vi "备用系数复合写入.vi"(8 "备用系数":cluster{"上限":dbl, "下限":dbl, "范围":dbl}, 9 "量程下拉列表":enum16{"低量程", "高量程"}(ring), 10 "测量模式":T1(ring), 11 "参数下拉列表":u16(ring) items=["总氮"=2]) -> ()   [LabVIEW 2016, in "斯坦道通用流路CODmn.lvlib"]
uses:
  <vilib>/Utility/miscctls.llb/LVPointTypeDef.ctl
panel:
  in  "读取":bool
  in  "一键写入":bool=TRUE
  out "连接的字符串":string
  in  "关闭":bool
  in  "写入":bool
  # "请选择要写入的参数"
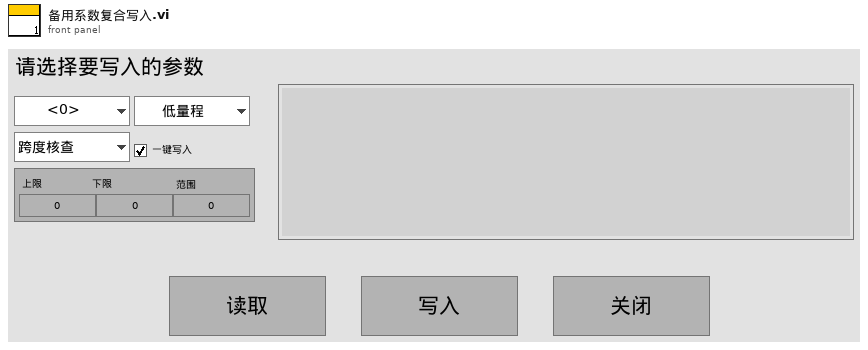
[diagram p1: front panel]
types:
  T1 = enum16{"跨度核查", "水样测量", "零点核查", "标样核查", "加标回收", "快捷测试", "空白校准", "标样校准"}
  T2 = typedef "LVPointTypeDef.ctl" = cluster{"Horizontal":i16, "Vertical":i16}
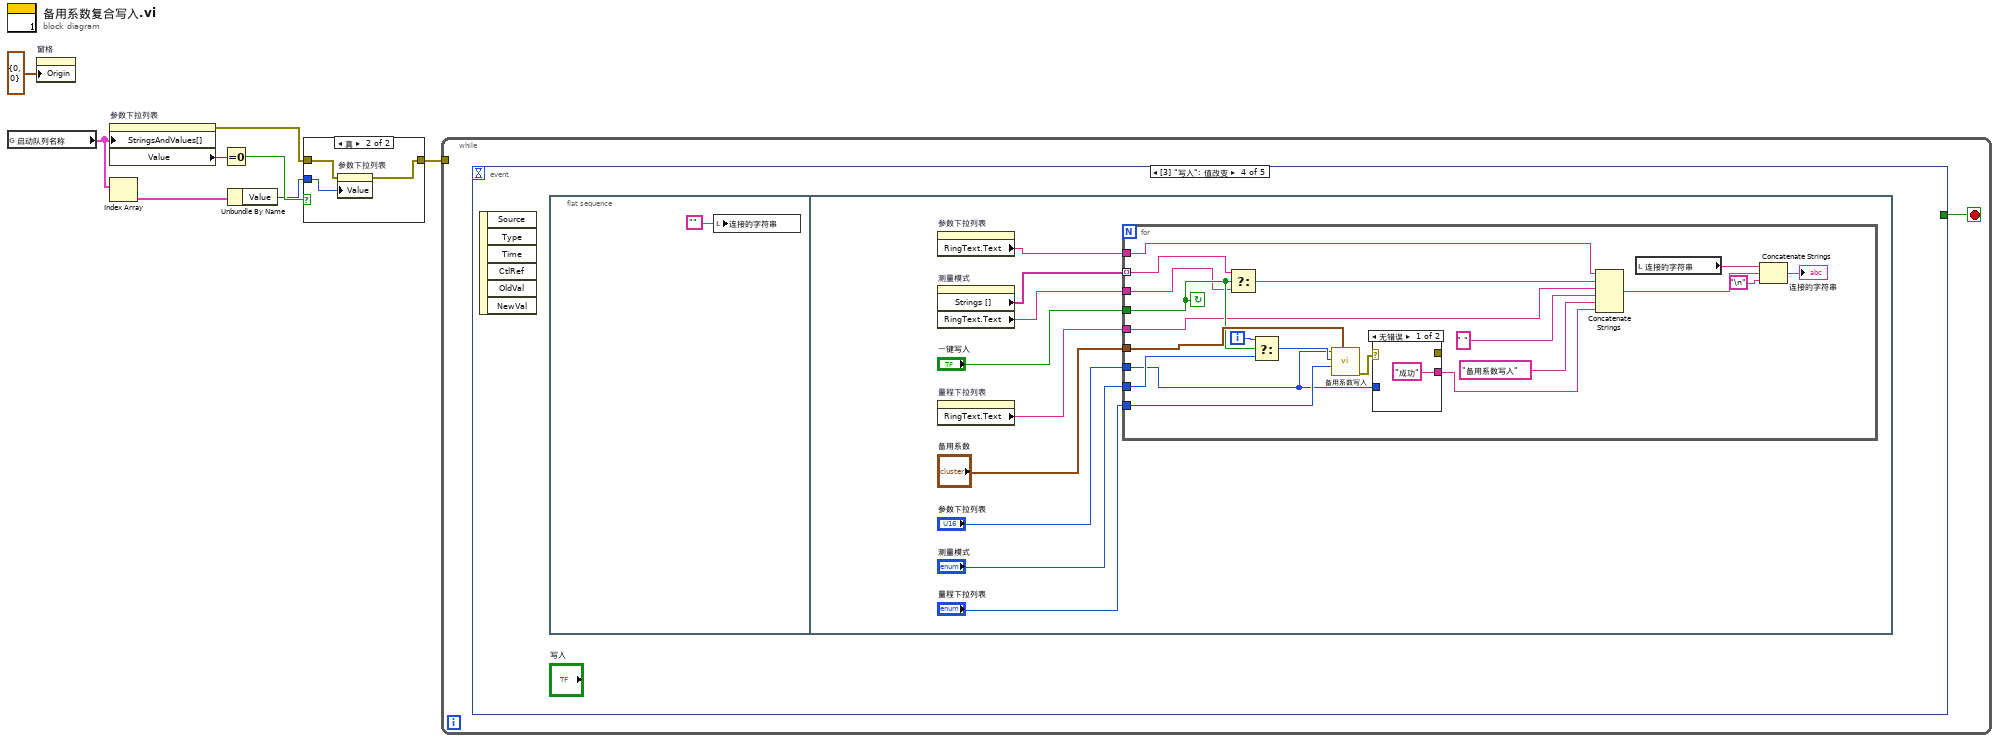
[diagram p0: block diagram]
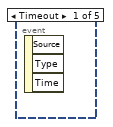
[diagram p3: hidden frame]
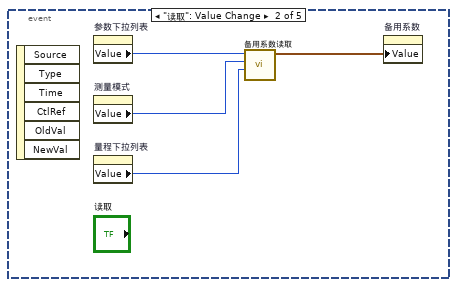
[diagram p4: hidden frame]
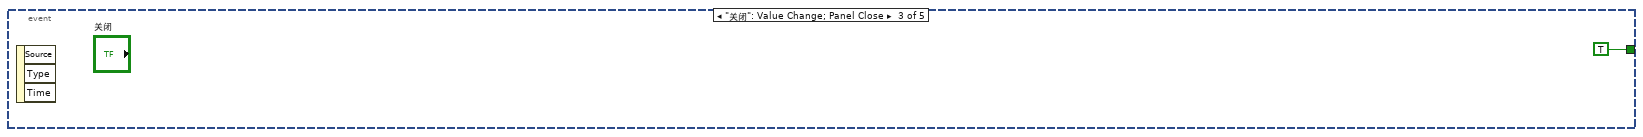
[diagram p5: hidden frame]
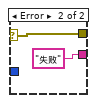
[diagram p6: hidden frame]
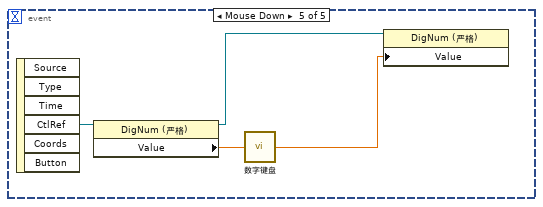
[diagram p7: hidden frame]
diagram:
  n1 = global read "model config var.vi" "启动队列名称"() -> (w3:cluster{"String":string, "Value":u16}[])
  n2 = property on="窗格" class="Pane"("Origin"=T2 {"Horizontal"=0, "Vertical"=0} ("原点")) -> ()  [unwired: 2 in, 2 out]
  n3 = property on="参数下拉列表" class="Ring (严格)"("StringsAndValues[]"=w3) -> (error out=w5:errorcluster, "Value"=w7:u16)  [unwired: 2 in, 1 out]
  n4 = Index Array(array=w3) -> (element=w2:cluster{"String":string, "Value":u16})  [unwired: 1 in]
  n5 = Equal To 0?(x=w7) -> (x = 0?=w6:bool)
  n6 = Unbundle By Name(w2) -> ("Value"=w1:u16)
  n7 = case shown="真" w6 {
    tunnel: w5 -> [w9 w12]
    tunnel: [w9 w11] -> w4
    tunnel: w1 -> [_ w10]
    frame False {
    }
    frame True {
      n8 = property on="参数下拉列表" class="Ring (严格)"(error in=w12, "Value"=w10) -> (error out=w11:errorcluster)  [unwired: 1 in, 1 out]
    }
  }
  n9 = while {
    tunnel: w4 -> [_]
    stop <- w13 stop-if-true
    n10 = event shown="[3] \"写入\": 值改变" {
      selector: _ -> [_ _ _ _ _]
      dyn-events: _ -> [_ _ _ _ _]
      timeout: _ -> [_ _ _ _ _]
      tunnel: [_ _ TRUE _ _] -> w13
      event Timeout {
        n11 = event-data() -> ()  [unwired: 1 in, 3 out]
      }
      event "读取": Value Change {
        n12 = event-data() -> ()  [unwired: 1 in, 6 out]
        n13 = property on="参数下拉列表" class="Ring (严格)"() -> ("Value"=w17:u16)  [unwired: 2 in, 2 out]
        n14 = property on="测量模式" class="Enum (严格)"() -> ("Value"=w16:T1)  [unwired: 2 in, 2 out]
        n15 = property on="量程下拉列表" class="Enum (严格)"() -> ("Value"=w15:enum16{"低量程", "高量程"})  [unwired: 2 in, 2 out]
        n16 = call "备用系数读取.vi"("量程"=w15, "测量模式"=w16, "测量参数"=w17) -> ("备用系数"=w14:cluster{"上限":dbl, "下限":dbl, "范围":dbl})  [unwired: 7 in, 1 out]
        n17 = property on="备用系数" class="Clust (严格)"("Value"=w14) -> ()  [unwired: 2 in, 2 out]
      }
      event "关闭": Value Change; Panel Close {
        n18 = event-data() -> ()  [unwired: 1 in, 3 out]
      }
      event "写入": Value Change {
        n19 = event-data() -> ()  [unwired: 1 in, 6 out]
        n20 = flat-sequence {
          frame #0 {
            n21 = local write "连接的字符串"("") -> ()
          }
          frame #1 {
            n22 = property on="参数下拉列表" class="Ring (严格)"() -> ("RingText.Text"=w21:string)  [unwired: 2 in, 2 out]
            n23 = property on="测量模式" class="Enum (严格)"() -> ("Strings []"=w25:string[], "RingText.Text"=w24:string)  [unwired: 2 in, 2 out]
            n24 = property on="量程下拉列表" class="Enum (严格)"() -> ("RingText.Text"=w20:string)  [unwired: 2 in, 2 out]
            n25 = for {
              tunnel: "备用系数" -> [w48]
              tunnel: "参数下拉列表" -> [w29]
              tunnel: "量程下拉列表" -> [w47]
              tunnel: w25 -> [w41] mode=indexing
              tunnel: w24 -> [w40]
              tunnel: "一键写入" -> [w42]
              tunnel: "测量模式" -> [w44]
              tunnel: w21 -> [w32]
              tunnel: w20 -> [w30]
              i -> [w45]
              stop <- w42 continue-if-true
              n26 = Select(t=w41, s=w42, f=w40) -> (s? t:f=w34:string)
              n27 = Select(t=w45, s=w42, f=w44) -> (s? t:f=w43:i32)
              n28 = call "备用系数写入.vi"("备用系数"=w48, "量程"=w47, "测量模式"=w43, "测量参数"=w29) -> ("error out"=w46:errorcluster)  [unwired: 6 in, 1 out]
              n29 = case shown="无错误" w46 {
                selector: w46 -> [_ w51]
                tunnel: [_ w51] -> _
                tunnel: ["成功" "失败"] -> w33
                tunnel: w29 -> [_ _]
                frame No Error {
                }
                frame Error {
                }
              }
              n30 = Concatenate Strings(w32, w34, w30, " " ("字符串"), "备用系数写入", w33) -> (w38:string)
              n31 = local read "连接的字符串"() -> (w35:string)
              n32 = Concatenate Strings(w35, w38, "\n") -> (→"连接的字符串":string)
            }
          }
        }
      }
      event "备用系数.上限", "备用系数.下限", "备用系数.范围": Mouse Down {
        n33 = event-data() -> ("CtlRef"=w55:refnum<vi>)  [unwired: 1 in, 5 out]
        n34 = property class="DigNum (严格)"(reference=w55) -> (reference out=w52:refnum<vi>, "Value"=w54:dbl)  [unwired: 1 in, 1 out]
        n35 = call "数字键盘.vi"("OldNumber"=w54) -> ("NewNumber"=w53:dbl)
        n36 = property class="DigNum (严格)"(reference=w52, "Value"=w53) -> ()  [unwired: 1 in, 2 out]
      }
    }
  }
